vi "Add Data Channels.vi"(8 "error in (no error)":errorcluster, 10 "Framework Configuration":refnum<class "Framework Configuration.lvclass">, 11 "Item Ref in":T1 format="%.0x") -> (0 "error out":errorcluster, 3 "Item Ref out":T1 format="%.0x")   [LabVIEW 2024, in "DSF System Explorer.lvlib"]
uses:
  DSF System Explorer.lvlib
  <vilib>/NI VeriStand/Custom Device API/Custom Device Item Ref.ctl
  Includes/DSF Core.lvlibp/Classes/Configuration/Core/Framework/Framework Configuration.lvclass
  <vilib>/NI VeriStand/Custom Device API/Custom Device Channel Type.ctl
  <vilib>/NI VeriStand/Custom Device API/Custom Device Channel.ctl
  Shared/Data Channel Page GUID.vi
  Shared/DSF Shared.lvlib
  Includes/DSF Core.lvlibp/Classes/Configuration/Core/Group/Group Configuration.lvclass
  Includes/DSF Core.lvlibp/Classes/Configuration/Core/Plugin/Plugin Configuration.lvclass
  Includes/DSF Core.lvlibp/Classes/Configuration/Core/Thread/Thread Configuration.lvclass
  Includes/DSF Core.lvlibp/Classes/Configuration/Core/Transfer/Transfer Configuration.lvclass
  Includes/DSF Core.lvlibp/Classes/Configuration/Core/Core Configuration.lvclass
  <vilib>/NI VeriStand/Custom Device API/Custom Device API.lvlib
  C:/dev/git/custom-devices/niveristand-data-sharing-framework-custom-device/Includes/DSF Core.lvlibp/Classes/Configuration/Core/Core Configuration.lvclass
  C:/dev/git/custom-devices/niveristand-data-sharing-framework-custom-device/Includes/DSF Core.lvlibp/Classes/Configuration/Configuration.lvclass
  C:/dev/git/custom-devices/niveristand-data-sharing-framework-custom-device/Includes/DSF Core.lvlibp/Classes/Configuration/Core/Plugin/Plugin Configuration.lvclass
  C:/dev/git/custom-devices/niveristand-data-sharing-framework-custom-device/Includes/DSF Core.lvlibp/Classes/Configuration/Core/Thread/Thread Configuration.lvclass
  C:/dev/git/custom-devices/niveristand-data-sharing-framework-custom-device/Includes/DSF Core.lvlibp/Classes/Configuration/Core/Group/Group Configuration.lvclass
  C:/dev/git/custom-devices/niveristand-data-sharing-framework-custom-device/Includes/DSF Core.lvlibp/Classes/Configuration/Core/Transfer/Transfer Configuration.lvclass
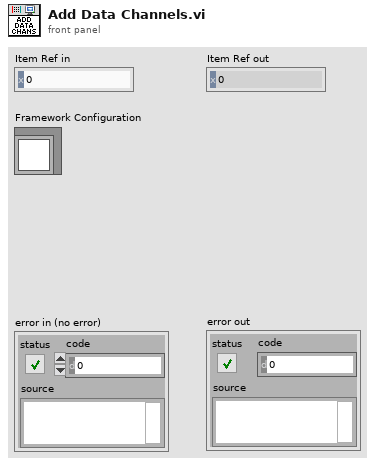
[diagram p1: front panel]
types:
  T1 = typedef "Custom Device API.lvlib/Custom Device Item Ref.ctl" = u64
  T2 = typedef "Custom Device API.lvlib/Custom Device Channel.ctl" = cluster{"Type":T3, "Units":string, "Default Value":dbl, "Faultable":bool, "Scalable":bool}
  T3 = typedef "Custom Device API.lvlib/Custom Device Channel Type.ctl" = enum16{"Input", "Output"}
  T4 = typedef "DSF Core.lvlibp/Plugin Configuration.lvclass/Core Plugin Configuration.ctl" = cluster{"name":string, "components":string[], "cycle timing":T5}
  T5 = typedef "DSF Core.lvlibp/DSF Timing Info.ctl" = cluster{"priority":u64, "decimation":u64, "offset":u64}
  T6 = typedef "DSF Core.lvlibp/DSF Settings Info.ctl" = cluster{"component":string, "values":cluster{"key":string, "value":string}[]}
  T7 = typedef "DSF Core.lvlibp/Thread Configuration.lvclass/Core Thread Configuration.ctl" = cluster{"processor":i32, "priority offset":i16}
  T8 = typedef "DSF Core.lvlibp/Group Configuration.lvclass/Core Group Configuration.ctl" = cluster{"name":string, "direction":T9, "cycle timing":T5, "timeout behavior":T10, "enable conversion":bool}
  T9 = typedef "DSF Core.lvlibp/DSF Direction.ctl" = enum8{"Tx", "Rx"}
  T10 = typedef "DSF Core.lvlibp/DSF Timeout Behavior.ctl" = enum8{"Increment Late Count", "Throw Error"}
  T11 = typedef "DSF Core.lvlibp/Transfer Configuration.lvclass/Core Transfer Configuration.ctl" = cluster{"name":string}
  T12 = typedef "DSF Core.lvlibp/Transfer Configuration.lvclass/Channel Configuration.ctl" = cluster{"configuration":T13, "component settings":T6[]}
  T13 = typedef "DSF Core.lvlibp/Channel Configuration.lvclass/Core Channel Configuration.ctl" = cluster{"name":string, "units":string, "engine data type":T14, "string data type":T14, "string offset":u64}
  T14 = typedef "DSF Core.lvlibp/DSF Data Type.ctl" = enum8{"Bool", "SGL", "DBL", "I8", "I16", "I32", "I64", "U8", "U16", "U32", "U64"}
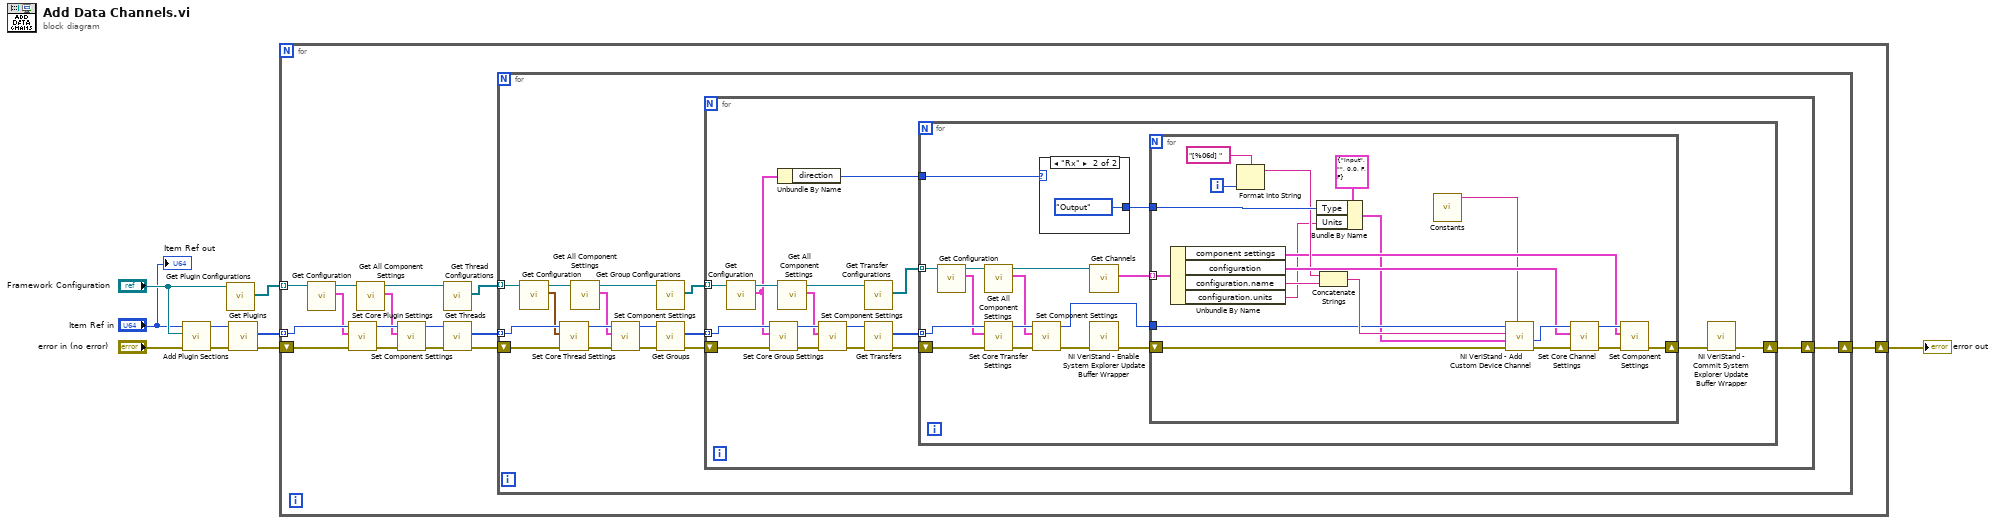
[diagram p0: block diagram]
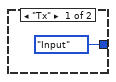
[diagram p2: hidden frame]
diagram:
  n1 = call "Add Plugin Sections.vi"("error in (no error)"="error in (no error)", "Framework Configuration"="Framework Configuration", "Item Ref in"="Item Ref in") -> ("error out"=w8:errorcluster, "Item Ref out"=w7:T1)  [unwired: 7 in]
  n2 = call "Get Plugin Configurations.vi"("Framework Configuration in"="Framework Configuration") -> ("Plugin Configurations"=w4:refnum<class "Plugin Configuration.lvclass">[])  [unwired: 8 in, 2 out]
  n3 = call "Get Plugins.vi"("error in (no error)"=w8, "Item Ref in"=w7) -> ("error out"=w6:errorcluster, "Plugin refs"=w5:T1[])  [unwired: 7 in, 1 out]
  n4 = for {
    tunnel: w5 -> [w16] mode=indexing
    tunnel: w4 -> [w18] mode=indexing
    shift-right: [w24] -> w9
    shift-left: w6 -> [w17]
    n5 = call "Get Configuration.vi"("Core Plugins Configuration in"=w18) -> ("configuration"=w15:T4, "Core Plugins Configuration out"=w12:refnum<class "Plugin Configuration.lvclass">)  [unwired: 8 in, 1 out]
    n6 = call "Set Core Plugin Settings.vi"("error in (no error)"=w17, "plugin configuration"=w15, "Item Ref in"=w16) -> ("error out"=w14:errorcluster, "Item Ref out"=w13:T1)  [unwired: 7 in]
    n7 = call "Get All Component Settings.vi"("Runtime Configuration in"=w12) -> ("component settings"=w11:T6[], "Runtime Configuration out"=w10:refnum<class "Plugin Configuration.lvclass">)  [unwired: 8 in, 1 out]
    n8 = call "Set Component Settings.vi"("error in (no error)"=w14, "component settings"=w11, "Item Ref in"=w13) -> ("error out"=w19:errorcluster, "Item Ref out"=w20:T1)  [unwired: 7 in]
    n9 = call "Get Thread Configurations.vi"("Plugin Configuration in"=w10) -> ("Thread Configurations"=w23:refnum<class "Thread Configuration.lvclass">[])  [unwired: 8 in, 2 out]
    n10 = call "Get Threads.vi"("error in (no error)"=w19, "Item Ref in"=w20) -> ("error out"=w22:errorcluster, "Plugin refs"=w21:T1[])  [unwired: 7 in, 1 out]
    n11 = for {
      tunnel: w21 -> [w33] mode=indexing
      shift-right: [w37] -> w24
      shift-left: w22 -> [w34]
      tunnel: w23 -> [w35] mode=indexing
      n12 = call "Get Configuration.vi"("Core Threads Configuration in"=w35) -> ("configuration"=w31:T7, "Core Threads Configuration out"=w32:refnum<class "Thread Configuration.lvclass">)  [unwired: 8 in, 1 out]
      n13 = call "Set Core Thread Settings.vi"("error in (no error)"=w34, "thread configuration"=w31, "Item Ref in"=w33) -> ("error out"=w30:errorcluster, "Item Ref out"=w29:T1)  [unwired: 7 in]
      n14 = call "Get All Component Settings.vi"("Runtime Configuration in"=w32) -> ("component settings"=w25:T6[], "Runtime Configuration out"=w26:refnum<class "Thread Configuration.lvclass">)  [unwired: 8 in, 1 out]
      n15 = call "Set Component Settings.vi"("error in (no error)"=w30, "component settings"=w25, "Item Ref in"=w29) -> ("error out"=w27:errorcluster, "Item Ref out"=w28:T1)  [unwired: 7 in]
      n16 = call "Get Group Configurations.vi"("Thread Configuration in"=w26) -> ("Group Configurations"=w36:refnum<class "Group Configuration.lvclass">[])  [unwired: 8 in, 2 out]
      n17 = call "Get Groups.vi"("error in (no error)"=w27, "Plugin Ref in"=w28) -> ("error out"=w39:errorcluster, "Group refs"=w38:T1[])  [unwired: 7 in, 1 out]
      n18 = for {
        shift-right: [w53] -> w37
        shift-left: w39 -> [w50]
        tunnel: w38 -> [w49] mode=indexing
        tunnel: w36 -> [w44] mode=indexing
        n19 = call "Get Configuration.vi"("Core Groups Configuration in"=w44) -> ("configuration"=w40:T8, "Core Groups Configuration out"=w43:refnum<class "Group Configuration.lvclass">)  [unwired: 8 in, 1 out]
        n20 = call "Set Core Group Settings.vi"("error in (no error)"=w50, "group configuration"=w40, "Item Ref in"=w49) -> ("error out"=w48:errorcluster, "Item Ref out"=w47:T1)  [unwired: 7 in]
        n21 = Unbundle By Name(w40) -> ("direction"=w51:T9)
        n22 = call "Get All Component Settings.vi"("Runtime Configuration in"=w43) -> ("component settings"=w42:T6[], "Runtime Configuration out"=w41:refnum<class "Group Configuration.lvclass">)  [unwired: 8 in, 1 out]
        n23 = call "Set Component Settings.vi"("error in (no error)"=w48, "component settings"=w42, "Item Ref in"=w47) -> ("error out"=w46:errorcluster, "Item Ref out"=w45:T1)  [unwired: 7 in]
        n24 = call "Get Transfer Configurations.vi"("Group Configuration in"=w41) -> ("Transfer Configurations"=w52:refnum<class "Transfer Configuration.lvclass">[])  [unwired: 8 in, 2 out]
        n25 = call "Get Transfers.vi"("error in (no error)"=w46, "Group Ref in"=w45) -> ("error out"=w55:errorcluster, "Transfer refs"=w54:T1[])  [unwired: 7 in, 1 out]
        n26 = for {
          shift-right: [w56] -> w53
          shift-left: w55 -> [w72]
          tunnel: w54 -> [w70] mode=indexing
          tunnel: w51 -> [w59]
          tunnel: w52 -> [w71] mode=indexing
          n27 = call "Get Configuration.vi"("Core Transfers Configuration in"=w71) -> ("configuration"=w69:T11, "Core Transfers Configuration out"=w65:refnum<class "Transfer Configuration.lvclass">)  [unwired: 8 in, 1 out]
          n28 = call "Get All Component Settings.vi"("Runtime Configuration in"=w65) -> ("component settings"=w64:T6[], "Runtime Configuration out"=w63:refnum<class "Transfer Configuration.lvclass">)  [unwired: 8 in, 1 out]
          n29 = call "Set Core Transfer Settings.vi"("error in (no error)"=w72, "transfer configuration"=w69, "Item Ref in"=w70) -> ("error out"=w68:errorcluster, "Item Ref out"=w67:T1)  [unwired: 7 in]
          n30 = call "Set Component Settings.vi"("error in (no error)"=w68, "component settings"=w64, "Item Ref in"=w67) -> ("error out"=w66:errorcluster, "Item Ref out"=w58:T1)  [unwired: 7 in]
          n31 = case shown="\"Rx\"" w59 {
            tunnel: [Custom_Device_Channel_Type."Input" ("Type") Custom_Device_Channel_Type."Output" ("Type")] -> w62
            frame "Tx" {
            }
            frame "Rx" {
            }
          }
          n32 = call "Get Channels.vi"("Transfer Configuration in"=w63) -> ("channels"=w60:T12[])  [unwired: 8 in, 2 out]
          n33 = call "NI VeriStand - Enable System Explorer Update Buffer Wrapper.vi"("error in"=w66) -> ("error out"=w57:errorcluster)  [unwired: 10 in]
          n34 = for {
            tunnel: w58 -> [w88]
            tunnel: w62 -> [w91]
            tunnel: w60 -> [w85] mode=indexing
            shift-right: [w77] -> w61
            shift-left: w57 -> [w87]
            i -> [w80]
            n35 = Unbundle By Name(w85) -> ("component settings"=w76:T6[], "configuration"=w83:T13, "configuration.name"=w82:string, "configuration.units"=w74:string)
            n36 = Format Into String(format string="[%06d] ", w80) -> (resulting string=w81:string)  [unwired: 2 in, 1 out]
            n37 = Bundle By Name(cluster=T2 {"Type"=enum."Input", "Units"="", "Default Value"=0.0, "Faultable"=FALSE, "Scalable"=FALSE} ("Channel"), "Type"=w91, "Units"=w74) -> (w75:T2)
            n38 = Concatenate Strings(w81, w82) -> (w90:string)
            n39 = call-poly "Constants.vi"() -> ("Status GUID"=w73:string)  [unwired: 11 in]
            n40 = call <vilib>:"NI VeriStand - Add Custom Device Channel.vi"("GUID (Default Channel)"=w73, "error in (no error)"=w87, "Channel"=w75, "Channel Name"=w90, "Parent Ref in"=w88) -> ("error out"=w86:errorcluster, "Channel Ref"=w84:T1)  [unwired: 3 in, 2 out]
            n41 = call "Set Core Channel Settings.vi"("error in (no error)"=w86, "channel configuration"=w83, "Item Ref in"=w84) -> ("error out"=w79:errorcluster, "Item Ref out"=w78:T1)  [unwired: 7 in]
            n42 = call "Set Component Settings.vi"("error in (no error)"=w79, "component settings"=w76, "Item Ref in"=w78) -> ("error out"=w77:errorcluster)  [unwired: 7 in, 1 out]
          }
          n43 = call "NI VeriStand - Commit System Explorer Update Buffer Wrapper.vi"("error in"=w61) -> ("error out"=w56:errorcluster)  [unwired: 10 in]
        }
      }
    }
  }
  "error out" <- w9
  "Item Ref out" <- "Item Ref in"
